vi "Read sync enable.vi"(8 "error in (no error)":errorcluster, 11 "Shared Memory configuration in":refnum<class "Shared Memory configuration.lvclass">) -> (0 "error out":errorcluster, 2 "sync enable":bool, 3 "Shared Memory configuration out":refnum<class "Shared Memory configuration.lvclass">)   [LabVIEW 2013, in "Shared Memory configuration.lvclass"]
uses:
  Shared Memory configuration.lvclass
  Shared Memory configuration.lvclass/Shared Memory configuration.ctl
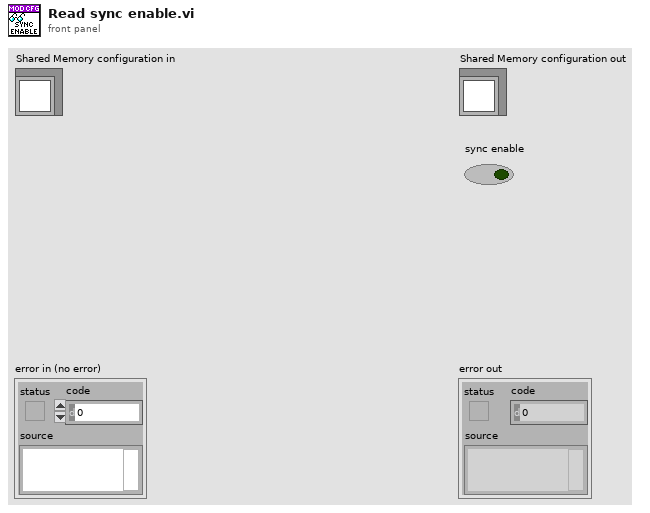
[diagram p1: front panel]
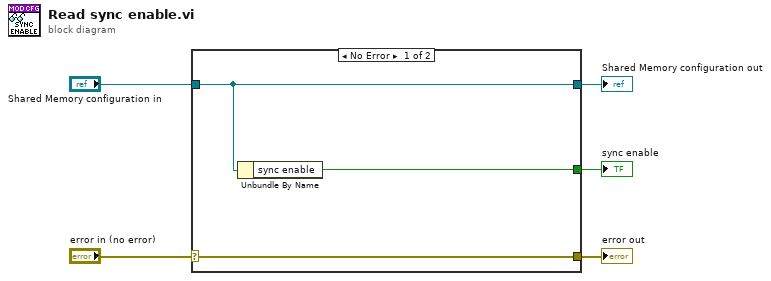
[diagram p0: block diagram]
diagram:
  n1 = case shown="No Error" "error in (no error)" {
    selector: "error in (no error)" -> [w8 w9]
    tunnel: [w8 w9] -> w4
    tunnel: [w7 w10] -> w2
    tunnel: "Shared Memory configuration in" -> [w7 w10]
    tunnel: [w6 _] -> w1
    frame No Error {
      n2 = Unbundle By Name(w7) -> ("sync enable"=w6:bool)
    }
    frame Error {
    }
  }
  "error out" <- w4
  "Shared Memory configuration out" <- w2
  "sync enable" <- w1
